vi "ping.vi"(8 "error in (no error)":errorcluster, 11 "TCP in":refnum<class "TCP.lvclass">) -> (0 "error out":errorcluster, 2 "Ping OK":bool, 3 "TCP out":refnum<class "TCP.lvclass">)   [LabVIEW 2021, in "TCP.lvclass"]
uses:
  TCP.lvclass
  D:/my_projects/projects/Algorithms/Labview/21/Master CR/Master CR.lvclass
  Master CR.lvclass/Master CR.ctl
  Param/TCP Param/TCP Param.lvclass
  Param/TCP Param/TCP Param.lvclass/TCP Param.ctl
  Master CR.lvclass
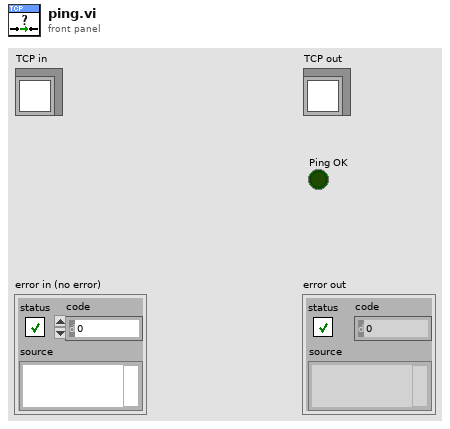
[diagram p1: front panel]
types:
  T1 = cluster{"Remote IP Address":string, "Remote Port":u16}
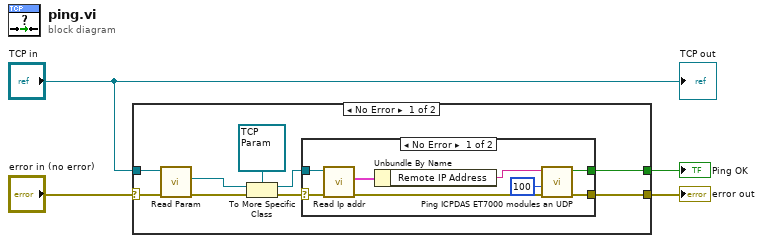
[diagram p0: block diagram]
diagram:
  n1 = case shown="No Error" "error in (no error)" {
    selector: "error in (no error)" -> [w10 w23]
    tunnel: [w6 w23] -> w3
    tunnel: "TCP in" -> [w13 _]
    tunnel: [w5 _] -> w1
    frame No Error {
      n2 = call "Read Param.vi"("error in (no error)"=w10, "MB_TCP in"=w13) -> ("error out"=w9:errorcluster, "Param"=w12:refnum<class "Param.lvclass">)  [unwired: 7 in, 1 out]
      n3 = To More Specific Class(target class=refnum<class "TCP Param.lvclass"> refnum ("Param.lvlib:TCP Param.lvclass"), reference=w12, error in=w9) -> (specific class reference=w7:refnum<class "TCP Param.lvclass">, error out=w8:errorcluster)
      n4 = case shown="No Error" w8 {
        selector: w8 -> [w21 w22]
        tunnel: w7 -> [w20 _]
        tunnel: [w16 w22] -> w6
        tunnel: [w15 _] -> w5
        frame No Error {
          n5 = call "Read Ip addr.vi"("error in (no error)"=w21, "MBParam in"=w20) -> ("error out"=w19:errorcluster, "IP address"=w18:T1)  [unwired: 7 in, 1 out]
          n6 = Unbundle By Name(w18) -> ("Remote IP Address"=w17:string)
          n7 = call "Ping ICPDAS ET7000 modules an UDP.vi"("error in (no error)"=w19, "timeout ms (100)"=100 ("timeout ms (200)"), "IP addr"=w17) -> ("error out"=w16:errorcluster, "OK"=w15:bool)  [unwired: 7 in]
        }
        frame Error {
        }
      }
    }
    frame Error {
    }
  }
  "error out" <- w3
  "Ping OK" <- w1
  "TCP out" <- "TCP in"
